vi "Build Private Data.vi"(6 "Wiring Spec":T2, 8 "error in (no error)":errorcluster, 10 "References":T1) -> (0 "error out":errorcluster)   [LabVIEW 2023, in "Message Maker.lvclass"]
doc: "Clears out the private data of the message and adds the needed data elements\n\nAuthor: Derek Trepanier\nCopyright: MGI 2015"
uses:
  Message Maker.lvclass
  Wiring Spec.ctl
  Connector Pane Position.ctl
  Scripting Refs.ctl
  <vilib>/Utility/traverseref.llb/TRef TravTarget.ctl
  <vilib>/Utility/miscctls.llb/LVPositionTypeDef.ctl
  Message Maker.lvclass/Message Maker.ctl
  <vilib>/Utility/traverseref.llb/VI Scripting - Traverse.lvlib
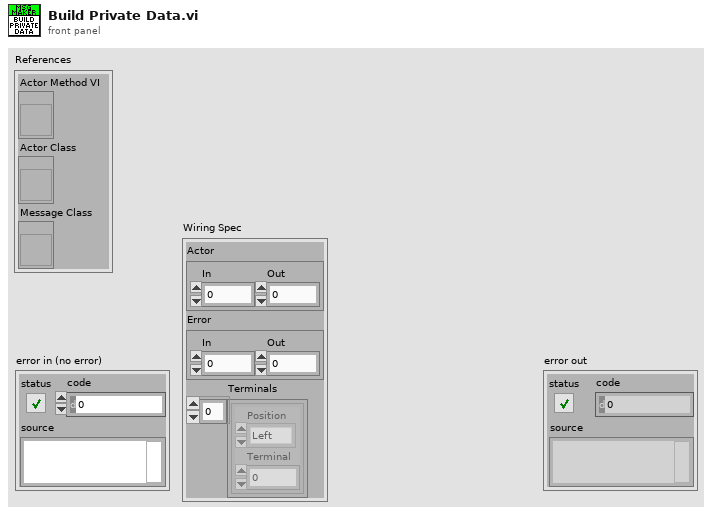
[diagram p1: front panel]
types:
  T1 = typedef "Message Maker.lvclass/Scripting Refs.ctl" = cluster{"Actor Method VI":refnum<vi>, "Actor Class":refnum<vi>, "Message Class":refnum<vi>}
  T2 = typedef "Message Maker.lvclass/Wiring Spec.ctl" = cluster{"Actor":cluster{"In":i32, "Out":i32}, "Error":cluster{"In":i32, "Out":i32}, "Terminals":cluster{"Position":T3, "Terminal":i32}[]}
  T3 = typedef "Message Maker.lvclass/Connector Pane Position.ctl" = enum16{"Left", "Top", "Bottom", "Right"}
  T4 = typedef "TRef TravTarget.ctl" = enum16{"FP", "BD", "Other"}
  T5 = typedef "LVPositionTypeDef.ctl" = cluster{"Left":i32, "Top":i32}
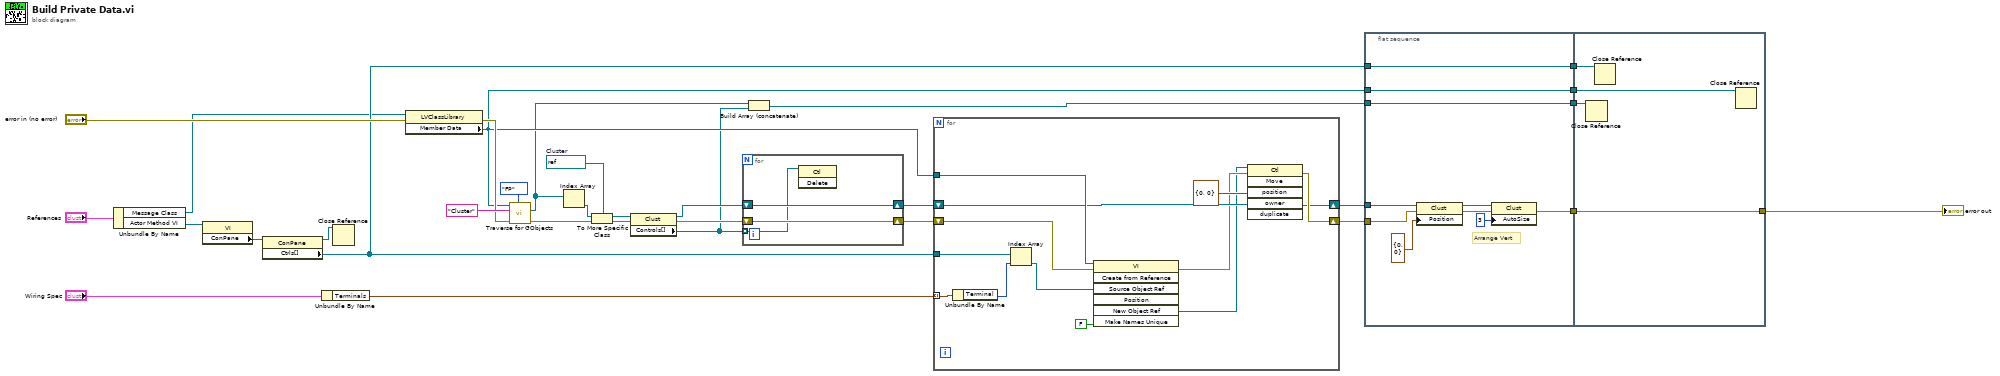
[diagram p0: block diagram]
diagram:
  w26 = refnum<vi> refnum  # Cluster
  n1 = Unbundle By Name("References") -> ("Message Class"=w11:refnum<vi>, "Actor Method VI"=w10:refnum<vi>)
  n2 = property class="VI"(reference=w10) -> ("ConPane"=w32:refnum<vi>)  [unwired: 1 in, 2 out]
  n3 = property class="ConPane"(reference=w32) -> (reference out=w24:refnum<vi>, "Ctrls[]"=w16:refnum<vi>[])  [unwired: 1 in, 1 out]
  n4 = Unbundle By Name("Wiring Spec") -> ("Terminals"=w13:cluster{"Position":T3, "Terminal":i32}[])
  n5 = Close Reference(reference=w24) -> ()  [unwired: 1 in, 1 out]
  n6 = property class="LVClassLibrary"(reference=w11, error in="error in (no error)") -> (error out=w29:errorcluster, "Member Data"=w23:refnum<vi>)  [unwired: 1 out]
  n7 = call <vilib>:"Traverse for GObjects.vi"("Traverse Target"=TRef_TravTarget."FP", "error in (no error)"=w29, "Class Name"="Cluster" ("name/order"), "VI Refnum"=w23) -> ("error out"=w25:errorcluster, "References"=w22:refnum<vi>[])  [unwired: 4 in, 2 out]
  n8 = Index Array(array=w22) -> (element=w28:refnum<vi>)  [unwired: 1 in]
  n9 = To More Specific Class(target class=w26, reference=w28, error in=w25) -> (specific class reference=w27:refnum<vi>, error out=w9:errorcluster)
  n10 = property class="Clust"(reference=w27, error in=w9) -> (reference out=w6:refnum<vi>, error out=w4:errorcluster, "Controls[]"=w1:refnum<vi>[])
  n11 = for {
    shift-right: [w34] -> w5
    shift-left: w6 -> [w34]
    shift-right: [w35] -> w3
    shift-left: w4 -> [w35]
    tunnel: w1 -> [w33] mode=indexing
    n12 = invoke class="Ctl" method="Delete"(reference=w33) -> ()  [unwired: 2 in, 3 out]
  }
  n13 = Build Array (concatenate)(w22, w1) -> (w2:refnum<vi>[])
  n14 = for {
    tunnel: w16 -> [w42]
    tunnel: w23 -> [w47]
    shift-right: [w46] -> w7
    shift-left: w3 -> [w40]
    shift-right: [w45] -> w8
    shift-left: w5 -> [w45]
    tunnel: w13 -> [w41] mode=indexing
    n15 = Unbundle By Name(w41) -> ("Terminal"=w39:i32)
    n16 = Index Array(array=w42, index=w39) -> (element=w38:refnum<vi>)
    n17 = invoke class="VI" method="Create from Reference"(reference=w47, error in=w40, "Source Object Ref"=w38, "Make Names Unique"=FALSE ("Make Names Unique (F)")) -> (error out=w43:errorcluster, "New Object Ref"=w37:refnum<vi>)  [unwired: 3 in, 5 out]
    n18 = invoke class="Ctl" method="Move"(reference=w37, error in=w43, "position"=T5 {"Left"=0, "Top"=0}, "owner"=w45) -> (error out=w46:errorcluster)  [unwired: 2 in, 5 out]
  }
  n19 = flat-sequence {
    tunnel: w8 -> [w57]
    tunnel: w7 -> [w52]
    tunnel: w23 -> [w49]
    tunnel: w2 -> [w51]
    tunnel: [w48] -> w19
    tunnel: [w49] -> w18
    tunnel: [w51] -> w17
    tunnel: w16 -> [w50]
    tunnel: [w50] -> w15
    tunnel: [w61] -> w20
    tunnel: w19 -> [w61]
    tunnel: w18 -> [w60]
    tunnel: w17 -> [w59]
    tunnel: w15 -> [w58]
    frame #0 {
      # "Arrange Vert"
      n20 = property class="Clust"(reference=w57, error in=w52, "Position"=T5 {"Left"=0, "Top"=0}) -> (reference out=w55:refnum<vi>, error out=w54:errorcluster)
      n21 = property class="Clust"(reference=w55, error in=w54, "AutoSize"=u32 3 ("Auto Sizing")) -> (error out=w48:errorcluster)  [unwired: 1 out]
    }
    frame #1 {
      n22 = Close Reference(reference=w59) -> ()  [unwired: 1 in, 1 out]
      n23 = Close Reference(reference=w58) -> ()  [unwired: 1 in, 1 out]
      n24 = Close Reference(reference=w60) -> ()  [unwired: 1 in, 1 out]
    }
  }
  "error out" <- w20
